vi "Color setting VI.vi"() -> (3 "Out":u32)   [LabVIEW 2016]
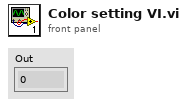
[diagram p1: front panel]
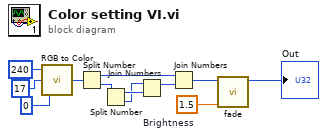
[diagram p0: block diagram]
diagram:
  w5 = 1.5  # Brightness
  n1 = call <vilib>:"RGB to Color.vi"("B"=u8 0, "G"=u8 17, "R"=u8 240) -> ("Color"=w9:u32)
  n2 = Split Number(x=w9) -> (hi(x)=w12:u16, lo(x)=w8:u16)
  n3 = Split Number(x=w8) -> (hi(x)=w10:u8, lo(x)=w7:u8)
  n4 = Join Numbers(hi=w7, lo=w10) -> ((hi.lo)=w11:u16)
  n5 = Join Numbers(hi=w12, lo=w11) -> ((hi.lo)=w6:u32)
  n6 = call "fade.vi"("Brightness"=w5, "In"=w6) -> ("Out"=→"Out":u32)  [unwired: 9 in]
